vi "State Vector Array.vi"(7 "QuWire in":refnum<class "QuWire.lvclass">) -> ()   [LabVIEW 2020]
uses:
  QuSim/QuWire/QuWire.lvclass
panel:
  out "Qubit Count":i32
  out "Basis States and State Vector":cluster{"State":i32, "Probability":cdb}[](array[cluster]) {"Probability" format="%#.6f"; "State" format="%07b"}
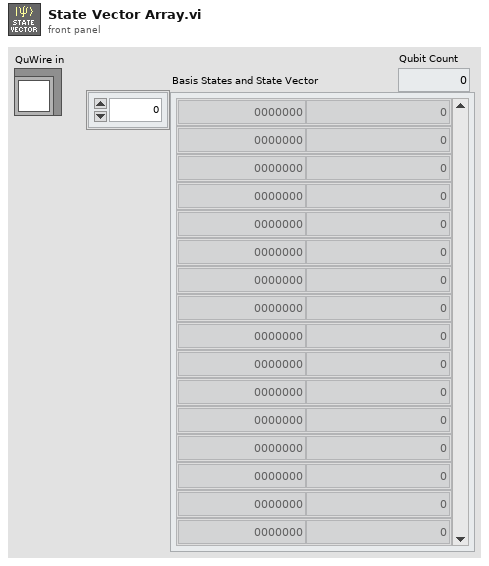
[diagram p1: front panel]
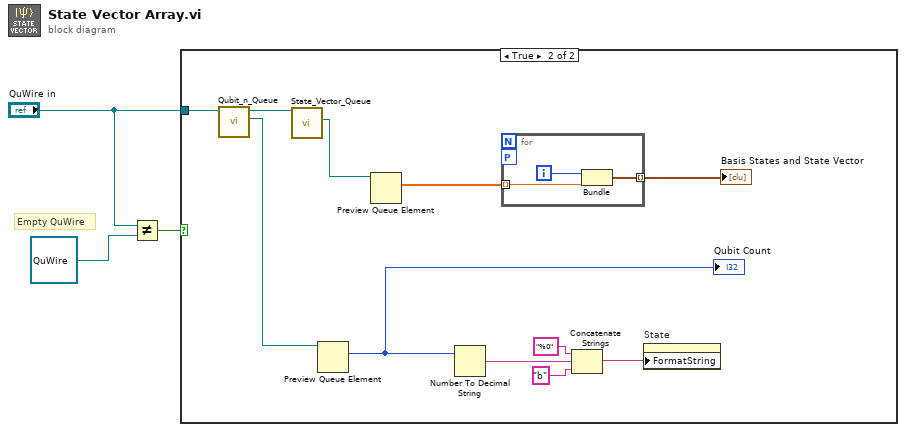
[diagram p0: block diagram]
diagram:
  # "Empty QuWire"
  n1 = Not Equal?(x="QuWire in", y=refnum<class "QuWire.lvclass"> refnum ("QuWire in")) -> (x != y?=w1:bool)
  n2 = case shown="True" w1 {
    tunnel: "QuWire in" -> [_ w14]
    frame False {
    }
    frame True {
      n3 = call "Qubit_n_Queue.vi"("QuWire in"=w14) -> ("Qubit n"=w6:refnum<queue>, "QuWire out"=w7:refnum<class "QuWire.lvclass">)  [unwired: 8 in, 1 out]
      n4 = call "State_Vector_Queue.vi"("QuWire in"=w7) -> ("State Vector Queue"=w13:refnum<queue>)  [unwired: 8 in, 2 out]
      n5 = Preview Queue Element(queue=w6) -> (element=w11:i32)  [unwired: 2 in, 3 out]
      "Qubit Count" <- w11
      n6 = Preview Queue Element(queue=w13) -> (element=w4:cdb[])  [unwired: 2 in, 3 out]
      n7 = Number To Decimal String(number=w11) -> (decimal integer string=w10:string)  [unwired: 1 in]
      n8 = for {
        tunnel: w4 -> [w16] mode=indexing
        tunnel: [w15] -> w12 mode=indexing
        workers-P: _ -> [_]
        i -> [w17]
        n9 = Bundle(w17, "Complex Matrix Element"=w16) -> (w15:cluster{i32, "Complex Matrix Element":cdb})  [unwired: 1 in]
      }
      "Basis States and State Vector" <- w12
      n10 = Concatenate Strings("%0" ("string"), w10, "b" ("string")) -> (w5:string)
      n11 = property on="State" class="DigNum (strict)"("FormatString"=w5) -> ()  [unwired: 2 in, 2 out]
    }
  }
